vi "RSZVB Delete Calibration Kit With Label.vi"(8 "error in (no error)":errorcluster {"code" format="%.0x"}, 9 "Calibration Kit Label (\"\")":string, 10 "Calibration Kit Name (\"\")":string, 11 "VISA session":refnum<visa-resource-name>) -> (0 "error out":errorcluster {"code" format="%.0x"}, 3 "dup VISA session":refnum<visa-resource-name>)   [LabVIEW 2011]
doc: "This VI deletes an imported or user-defined cal kit which is identified by its cal kit name and label.\n\nRemote-control command(s):\n[SENSe<Ch>:]CORRection:CKIT:LDELete '<ckit_name>', '<ckit_label>'"
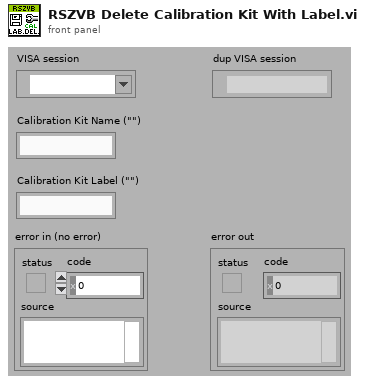
[diagram p1: front panel]
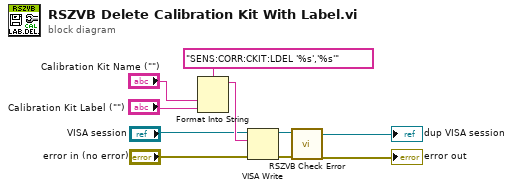
[diagram p0: block diagram]
diagram:
  n1 = Format Into String(format string="SENS:CORR:CKIT:LDEL '%s','%s'", "Calibration Kit Name (\"\")", "Calibration Kit Label (\"\")") -> (resulting string=w10:string)  [unwired: 2 in, 1 out]
  n2 = VISA Write(VISA resource name="VISA session", write buffer=w10, error in (no error)="error in (no error)") -> (VISA resource name out=w8:refnum<visa-resource-name>, error out=w9:errorcluster)  [unwired: 1 out]
  n3 = call "RSZVB Check Error.vi"("error in (no error)"=w9, "VISA session"=w8) -> ("error out"=→"error out":errorcluster, "dup VISA session"=→"dup VISA session":refnum<visa-resource-name>)  [unwired: 8 in]
